vi "S2C_VLFT10_Proc_FpButtSwitch.vi"(8 "Error In":errorcluster, 10 "State":T1 items=["SWITCH_STATE_NULL", "SWITCH_STATE_PRESSED", "SWITCH_STATE_RELEASED", "NUM_SWITCH_STATES"], 11 "Button":T2 items=["FPB_NONE", "FPB_POWER", "FPB_RECALL_SETTINGS", "FPB_SERVICE_MENU", "FPB_VOLUME", "FPB_BRIGHTNESS"]) -> (0 "Error Out":errorcluster, 3 "Pass?":bool)   [LabVIEW 2015]
uses:
  Fornax/VIs/PolyDriver/Typedefs/FrontPanelButtonId.ctl
  Fornax/VIs/PolyDriver/Typedefs/SwitchState.ctl
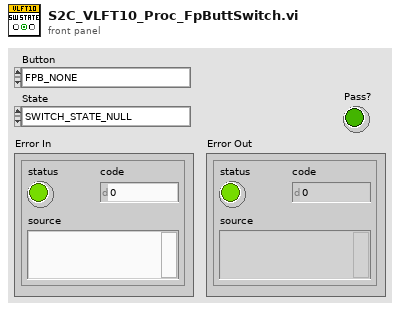
[diagram p1: front panel]
types:
  T1 = typedef "SwitchState.ctl" = i16
  T2 = typedef "FrontPanelButtonId.ctl" = i16
  T3 = cluster{"Partition":string, "Message":string, "M_ButtonId":T2, "M_SwitchState":T1}
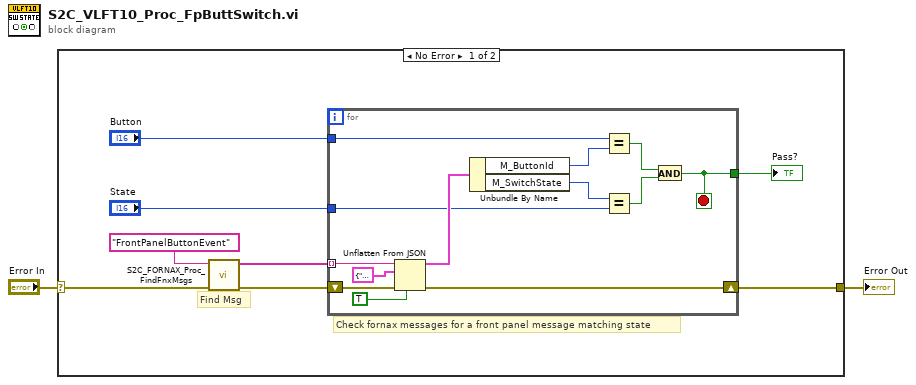
[diagram p0: block diagram]
diagram:
  n1 = case shown="No Error" "Error In" {
    selector: "Error In" -> [w7 w24]
    tunnel: [w6 w24] -> w2
    frame No Error {
      # "Find Msg"
      # "Check fornax messages for a front panel message matching state"
      n2 = call "S2C_FORNAX_Proc_FindFnxMsgs.vi"("Error In"=w7, "MsgName"="FrontPanelButtonEvent") -> ("Error Out"=w9:errorcluster, "Messages"=w8:string[])  [unwired: 8 in]
      n3 = for {
        tunnel: w8 -> [w19] mode=indexing
        tunnel: "Button" -> [w18]
        tunnel: "State" -> [w17]
        tunnel: [w14] -> w3
        shift-right: [w13] -> w6
        shift-left: w9 -> [w20]
        stop <- w14 stop-if-true
        n4 = Unflatten From JSON(JSON string=w19, type and defaults=T3 {"Partition"="", "Message"="", "M_ButtonId"=0, "M_SwitchState"=0}, default null elements? (F)=TRUE, error in (no error)=w20) -> (value=w21:T3, error out=w13:errorcluster)  [unwired: 3 in]
        n5 = Unbundle By Name(w21) -> ("M_ButtonId"=w12:T2, "M_SwitchState"=w11:T1)
        n6 = Equal?(x=w18, y=w12) -> (x = y?=w16:bool)
        n7 = Equal?(x=w11, y=w17) -> (x = y?=w15:bool)
        n8 = And(x=w16, y=w15) -> (x .and. y?=w14:bool)
      }
      "Pass?" <- w3
    }
    frame Error {
    }
  }
  "Error Out" <- w2
